vi "Event Driven State Machine.vi"() -> ()   [LabVIEW 2020]
uses:
  States.ctl
panel:
  out "Count":u32
  in  "Stop":bool
  in  "Start":bool
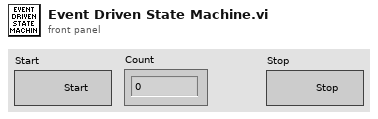
[diagram p1: front panel]
types:
  T1 = typedef "States.ctl" = enum16{"Initialize", "Wait for event", "Count Number", "Start", "Stop", "Shut Down"}
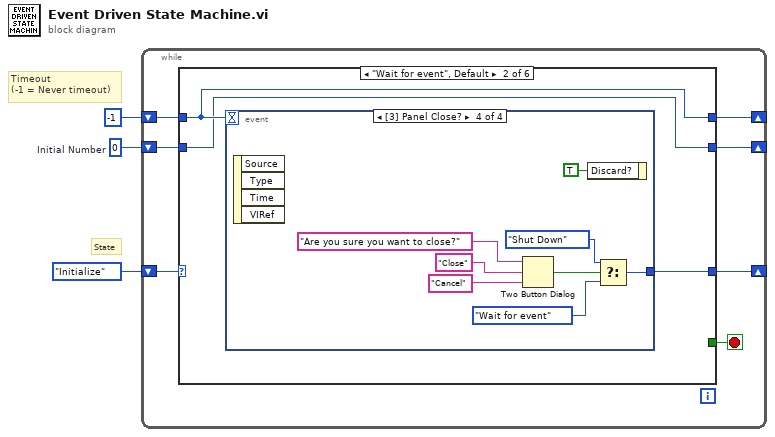
[diagram p0: block diagram]
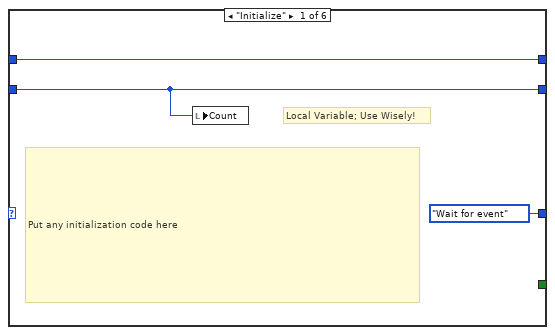
[diagram p2: hidden frame]
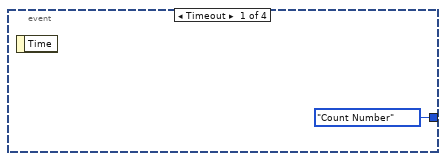
[diagram p3: hidden frame]
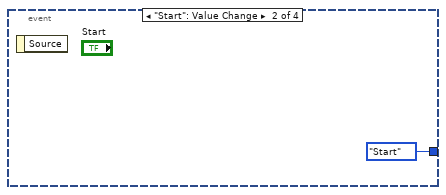
[diagram p4: hidden frame]
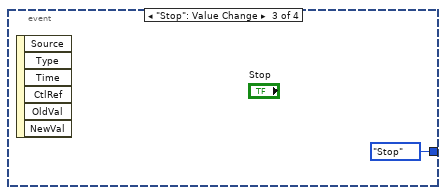
[diagram p5: hidden frame]
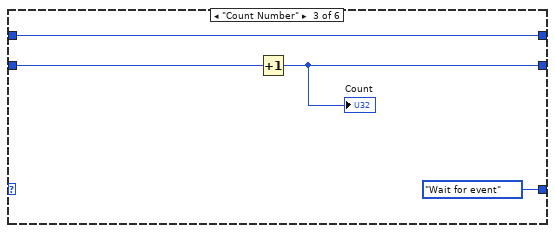
[diagram p6: hidden frame]
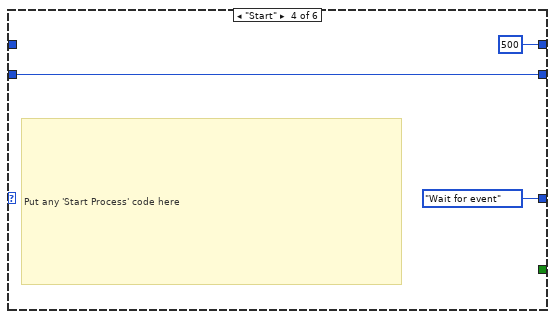
[diagram p7: hidden frame]
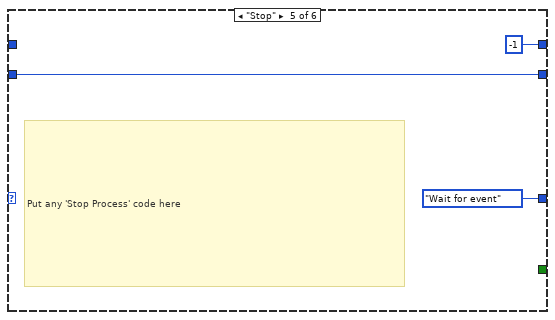
[diagram p8: hidden frame]
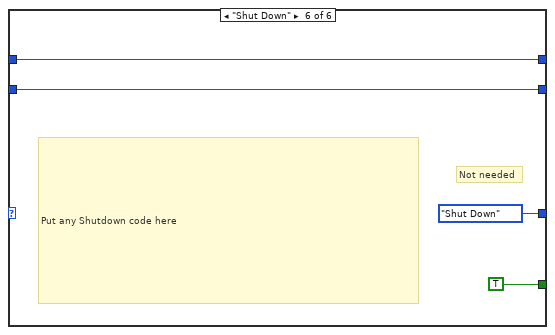
[diagram p9: hidden frame]
diagram:
  w1 = u32 0  # Initial Number
  # "State"
  # "Timeout\n(-1 = Never timeout)"
  n1 = while {
    shift-right: [w9] -> _
    shift-left: States."Initialize" ("States") -> [w4]
    shift-right: [w7] -> _
    shift-left: -1 -> [w10]
    shift-right: [w6] -> _
    shift-left: w1 -> [w5]
    stop <- w8 stop-if-true
    n2 = case shown="\"Wait for event\", Default" w4 {
      tunnel: w10 -> [w13 w15 w31 _ _ w39]
      tunnel: [States."Wait for event" ("States") w16 States."Wait for event" ("States") States."Wait for event" ("States") States."Wait for event" ("States") States."Shut Down" ("States")] -> w9
      tunnel: [_ _ _ _ _ TRUE] -> w8
      tunnel: [w13 w15 w31 500 -1 w39] -> w7
      tunnel: [w11 w14 w28 w32 w36 w38] -> w6
      tunnel: w5 -> [w11 w14 w29 w32 w36 w38]
      frame "Initialize" {
        # "Local Variable; Use Wisely!"
        # "Put any initialization code here"
        n3 = local write "Count"(w11) -> ()
      }
      frame "Wait for event", Default {
        n4 = event shown="[3] Panel Close?" {
          selector: _ -> [_ _ _ _]
          dyn-events: _ -> [_ _ _ _]
          timeout: w15 -> [_ _ _ _]
          tunnel: [States."Count Number" ("States") States."Start" ("States") States."Stop" ("States") w20] -> w16
          event Timeout {
            n5 = event-data() -> ()  [unwired: 1 in, 1 out]
          }
          event "Start": Value Change {
            n6 = event-data() -> ()  [unwired: 1 in, 1 out]
          }
          event "Stop": Value Change {
            n7 = event-data() -> ()  [unwired: 1 in, 6 out]
          }
          event Panel Close? {
            n8 = event-data() -> ()  [unwired: 1 in, 4 out]
            n9 = Two Button Dialog(message="Are you sure you want to close?", 1:"Cancel" ("F button name (\"Cancel\")"), 2:"Close" ("T button name (\"OK\")")) -> (T button?=w23:bool)
            n10 = event-data("Discard?"=TRUE) -> ()  [unwired: 1 in, 1 out]
            n11 = Select(t=States."Shut Down" ("States"), s=w23, f=States."Wait for event") -> (s? t:f=w20:T1)
          }
        }
      }
      frame "Count Number" {
        n12 = Increment(x=w29) -> (x+1=w28:u32)
        "Count" <- w28
      }
      frame "Start" {
        # "Put any 'Start Process' code here"
      }
      frame "Stop" {
        # "Put any 'Stop Process' code here"
      }
      frame "Shut Down" {
        # "Put any Shutdown code here"
        # "Not needed"
      }
    }
  }
